vi "write_ini_file.vi"() -> ()   [LabVIEW 2011]
uses:
  <vilib>/Utility/config.llb/Write Key (I32).vi
  <vilib>/Utility/config.llb/NI_LVConfig.lvlib
panel:
  out "key names":string[](array[string]) caption="键名"
  out "section exists?":bool caption="段存在？"
  out "found?":bool caption="已找到？"
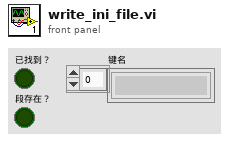
[diagram p1: front panel]
types:
  T1 = typedef "NI_LVConfig.lvlib/Config Data RefNum.ctl" = refnum<k1>
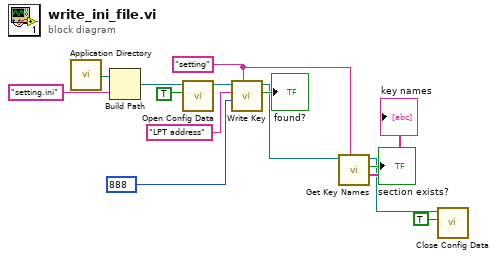
[diagram p0: block diagram]
diagram:
  w5 = "setting" ("section")
  n1 = call <vilib>:"Application Directory.vi"() -> ("Application Directory"=w14:path)
  n2 = Build Path(base path=w14, name or relative path="setting.ini" ("名称或相对路径")) -> (appended path=w12:path)
  n3 = call <vilib>:"Open Config Data.vi"("create file if necessary (T)"=TRUE, "configuration file path"=w12) -> ("refnum"=w10:T1)  [unwired: 7 in, 2 out]
  n4 = call-poly <vilib>:"Write Key.vi"("section"=w5, "value"=888, "key"="LPT address", "refnum"=w10) -> ("found?"=→"found?":bool, "refnum out"=w6:T1)  [unwired: 5 in, 1 out]
  n5 = call <vilib>:"Get Key Names.vi"("section"=w5, "refnum"=w6) -> ("key names"=→"key names":string[], "section exists?"=→"section exists?":bool, "refnum out"=w2:T1)  [unwired: 6 in, 1 out]
  n6 = call <vilib>:"Close Config Data.vi"("write file if changed (T)"=TRUE, "refnum"=w2) -> ()  [unwired: 8 in, 2 out]
